vi "Redundancy.vi"() -> ()   [LabVIEW 2013]
uses:
  Classes/OSSP_Problem.lvclass
  Classes/GanntChart_Class/Check Other Machines for Schedule Time.vi
  Classes/GanntChart_Class/Schedule Job.vi
  Classes/GanntChart_Class/Find Gaps on Particular Machine.vi
  Classes/GanntChart_Class/Increment Number of Jobs on Machine.vi
  Classes/GanntChart_Class/Operation to Machine Job Tuple.vi
  Classes/GanntChart_Class/Find Job On Other Machines.vi
  Classes/GanntChart.lvclass
panel:
  out "Processing Times":u16[][](array[numeric])
  out "Makespan 2":i32
  in  "Array 2":i32[](array[numeric])
  out "Makespan 1":i32
  in  "Array 1":i32[](array[numeric])
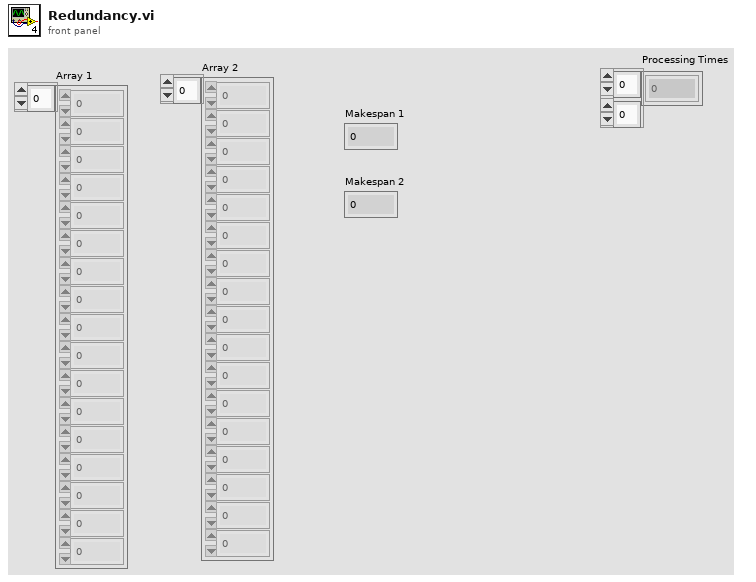
[diagram p1: front panel]
types:
  T1 = typedef "GanntChart_Element.ctl" = cluster{"Operation Number":i32, "Job Number":i32, "Start Time":i32, "Procesing Time":u16, "End Time":i32}
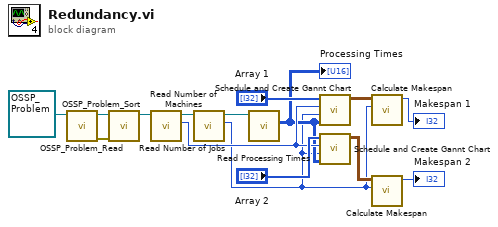
[diagram p0: block diagram]
diagram:
  n1 = call "OSSP_Problem_Read.vi"("OSSP_Problem.lvclass In"=refnum<class "OSSP_Problem.lvclass"> refnum ("OSSP_Problem.lvclass")) -> ("error out"=w13:errorcluster, "OSSP_Problem.lvclass Out"=w14:refnum<class "OSSP_Problem.lvclass">)  [unwired: 9 in]
  n2 = call "OSSP_Problem_Sort.vi"("error in (no error)"=w13, "OSSP_Problem.lvclass In"=w14) -> ("OSSP_Problem.lvclass Out"=w12:refnum<class "OSSP_Problem.lvclass">)  [unwired: 8 in, 1 out]
  n3 = call-dynamic "Read Number of Machines.vi"("OSSP_Problem in"=w12) -> ("Number of Machines"=w4:i32, "OSSP_Problem out"=w11:refnum<class "OSSP_Problem.lvclass">)  [unwired: 8 in, 1 out]
  n4 = call-dynamic "Read Number of Jobs.vi"("OSSP_Problem in"=w11) -> ("Number of Jobs"=w2:i32, "OSSP_Problem out"=w10:refnum<class "OSSP_Problem.lvclass">)  [unwired: 8 in, 1 out]
  n5 = call-dynamic "Read Processing Times.vi"("OSSP_Problem in"=w10) -> ("Processing Times"=w3:u16[][])  [unwired: 8 in, 2 out]
  "Processing Times" <- w3
  n6 = call "Schedule and Create Gannt Chart.vi"("Processing Times (Rows Mach.Cols Jobs)"=w3, "Number of Jobs"=w2, "Number of Machines"=w4, "Schedule"="Array 1") -> ("Gannt Chart Out"=w9:T1[][])  [unwired: 6 in, 1 out]
  n7 = call "Schedule and Create Gannt Chart.vi"("Processing Times (Rows Mach.Cols Jobs)"=w3, "Number of Jobs"=w2, "Number of Machines"=w4, "Schedule"="Array 2") -> ("Gannt Chart Out"=w6:T1[][])  [unwired: 6 in, 1 out]
  n8 = call "Calculate Makespan.vi"("Number of Jobs"=w2, "Gannt Chart In"=w9) -> ("Makespan"=→"Makespan 1":i32)  [unwired: 9 in]
  n9 = call "Calculate Makespan.vi"("Number of Jobs"=w2, "Gannt Chart In"=w6) -> ("Makespan"=→"Makespan 2":i32)  [unwired: 9 in]
